vi "ADCP_UI.vi"() -> ()   [LabVIEW 2017]
uses:
  Controls/ADCP_UI/ADCP_UI_Node_Requests.ctl
  Controls/ADCP_UI/ADCP_UI_Parameters.ctl
  Controls/ADCP_UI/ADCP_UI_Queues.ctl
  Controls/ADCP_UI/ADCP_UI_Continuous_Receiver_States.ctl
  Controls/ADCP_UI/ADCP_Queue_Receive_Log_Queue_Element.ctl
  Controls/Packet/Packet.ctl
  Controls/Packet/Packet_Direction.ctl
  Controls/Packet/Packet_Type.ctl
  Controls/Packet/Packet_Priority.ctl
  Controls/Data Packets/Data_Packet.ctl
  Controls/Data Packets/Parameter.ctl
  Controls/Data Packets/Parameter_Data_Type.ctl
  Controls/Data Packets/Data_Packet_Transmit_Mode.ctl
  ADCP_UI_Receive_List_Data_Packets.vi
panel:
  out "Node Requests":T1
  out "Receiver queue size":u32
  out "Receiver Queue Status":enum16{"OK", "EMPTY", "FULL"}(ring)
  out "Network Error Status":T2(ring)
  in  "Stop Application":bool
  in  "Receive Data Packet Log File Path":path
  in  "Transmit Data Packet Log File Path":path
  in  "Remove transmit list frame":bool
  in  "Add transmit list frame":bool
  in  "Transmit List Frame name":string(combo)
  out "Request frames":string[](array[string])
  in  "Remove request frame":bool
  in  "Add request frame":bool
  in  "Request Frame":string(combo)
  in  "Request frames from node":bool
  in  "Enable/disable node":bool
  in  "Get node status":bool
  in  "Reset nodes":bool
  in  "Node names":string(combo)="0"
  in  "Reset node":bool
  in  "Transmit List":string[][](table)
  in  "Receive List":string[][](table)
  in  "Load Symbol File":bool
  in  "Symbol File Path":path=path "F:/Projects/ADCP/LabVIEW/Symbol Files/default.csv"
  in  "Connect/Disconnect":bool
  in  "Baud rate":u32=38400
  in  "COM Port":refnum<visa-resource-name>="COM13"
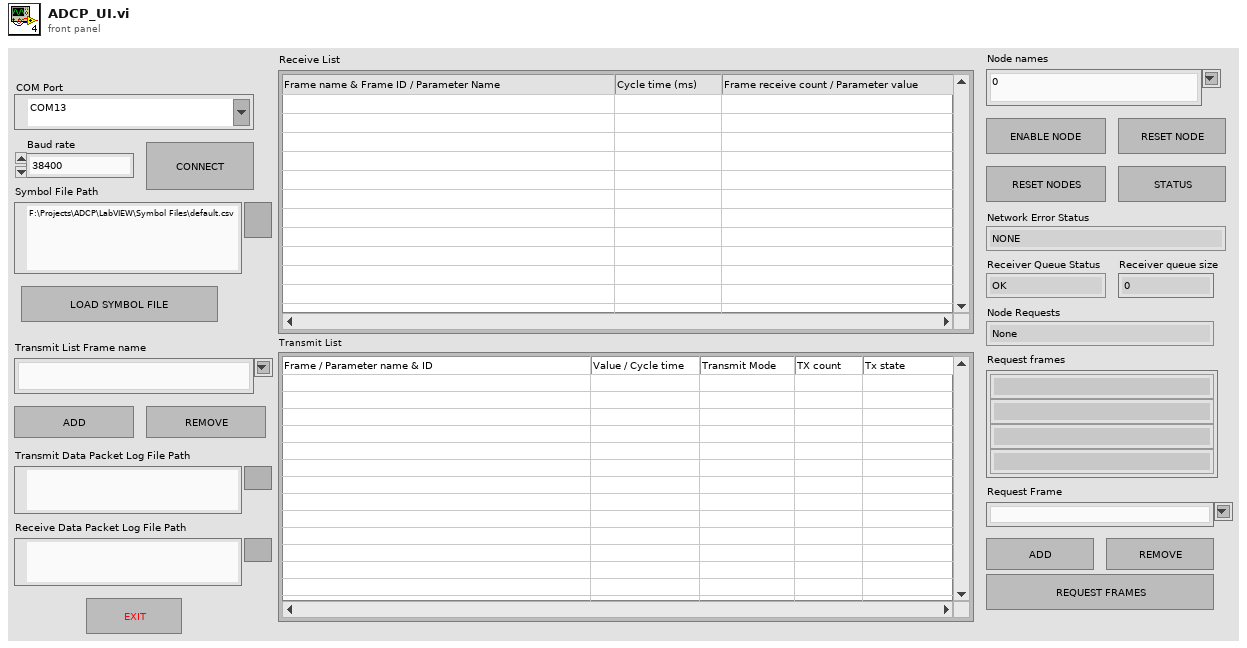
[diagram p1: front panel]
types:
  T1 = typedef "ADCP_UI_Node_Requests.ctl" = enum16{"None", "Open Connection RQST", "Open Connection ACK", "Close Connection RQST", "Close Connection ACK", "Sync/Reset RQST", "Sync/Reset ACK", "Error & Status RQST", "Error & Status ACK", "Remote Request RQST", "Remote Request ACK", "Timeout"}
  T2 = enum16{"NONE", "CONNECTION_ALREADY_OPEN", "CONNECTION_ALREADY_CLOSED", "INVALID_FRAME_REQUEST"}
  T3 = typedef "ADCP_UI_Parameters.ctl" = cluster{"COM Port":refnum<vi>, "Baud rate":refnum<vi>, "Symbol File Path":refnum<vi>, "Receive List":refnum<vi>, "Transmit List":refnum<vi>, "Node names":refnum<vi>, "Request Frame":refnum<vi>, "Request frames":refnum<vi>, "Transmit List Frame name":refnum<vi>, "Transmit Data Packet Log File Path":refnum<vi>, "Receive Data Packet Log File Path":refnum<vi>, "Loop 1 Resume Request":bool, "Loop 1 Pause Request":bool, "Loop 2 Resume Request":bool, "Loop 2 Pause Request":bool, "Loop 3 Resume Request":bool, "Loop 3 Pause Request":bool, "Loop 4 Resume Request":bool, "Loop 4 Pause Request":bool, "Loop 5 Resume Request":bool, "Loop 5 Pause Request":bool, "Loop 6 Resume Request":bool, "Loop 6 Pause Request":bool, "Loop 7 Resume Request":bool, "Loop 7 Pause Request":bool, "Loop 8 Resume Request":bool, "Loop 8 Pause Request":bool, "Exit":refnum<vi>, "Connect/Disconnect":refnum<vi>, "Load Symbol File":refnum<vi>, "Reset node":refnum<vi>, "Reset nodes":refnum<vi>, "Get node status":refnum<vi>, "Enable/disable node":refnum<vi>, "Request frames from node":refnum<vi>, "Remove request frame":refnum<vi>, "Add request frame":refnum<vi>, "Remove transmit list frame":refnum<vi>, "Add transmit list frame":refnum<vi>, "Receiver queue size":refnum<vi>, "Network Error Status":refnum<vi>, "Receiver Queue Status":refnum<vi>, "Node Requests":refnum<vi>, "Queues":T4}
  T4 = typedef "ADCP_UI_Queues.ctl" = cluster{"Continuous Receiver - Getter":refnum<queue>, "Continuous Receiver - Setter":refnum<queue>, "Receive Log":refnum<queue>, "Receive Table":refnum<queue>, "Receive List UI Table Updater":refnum<queue>, "Continuous Transmitter - Getter":refnum<queue>, "Continuous Transmitter - Setter":refnum<queue>, "Transmit Log":refnum<queue>, "Transmit Table":refnum<queue>}
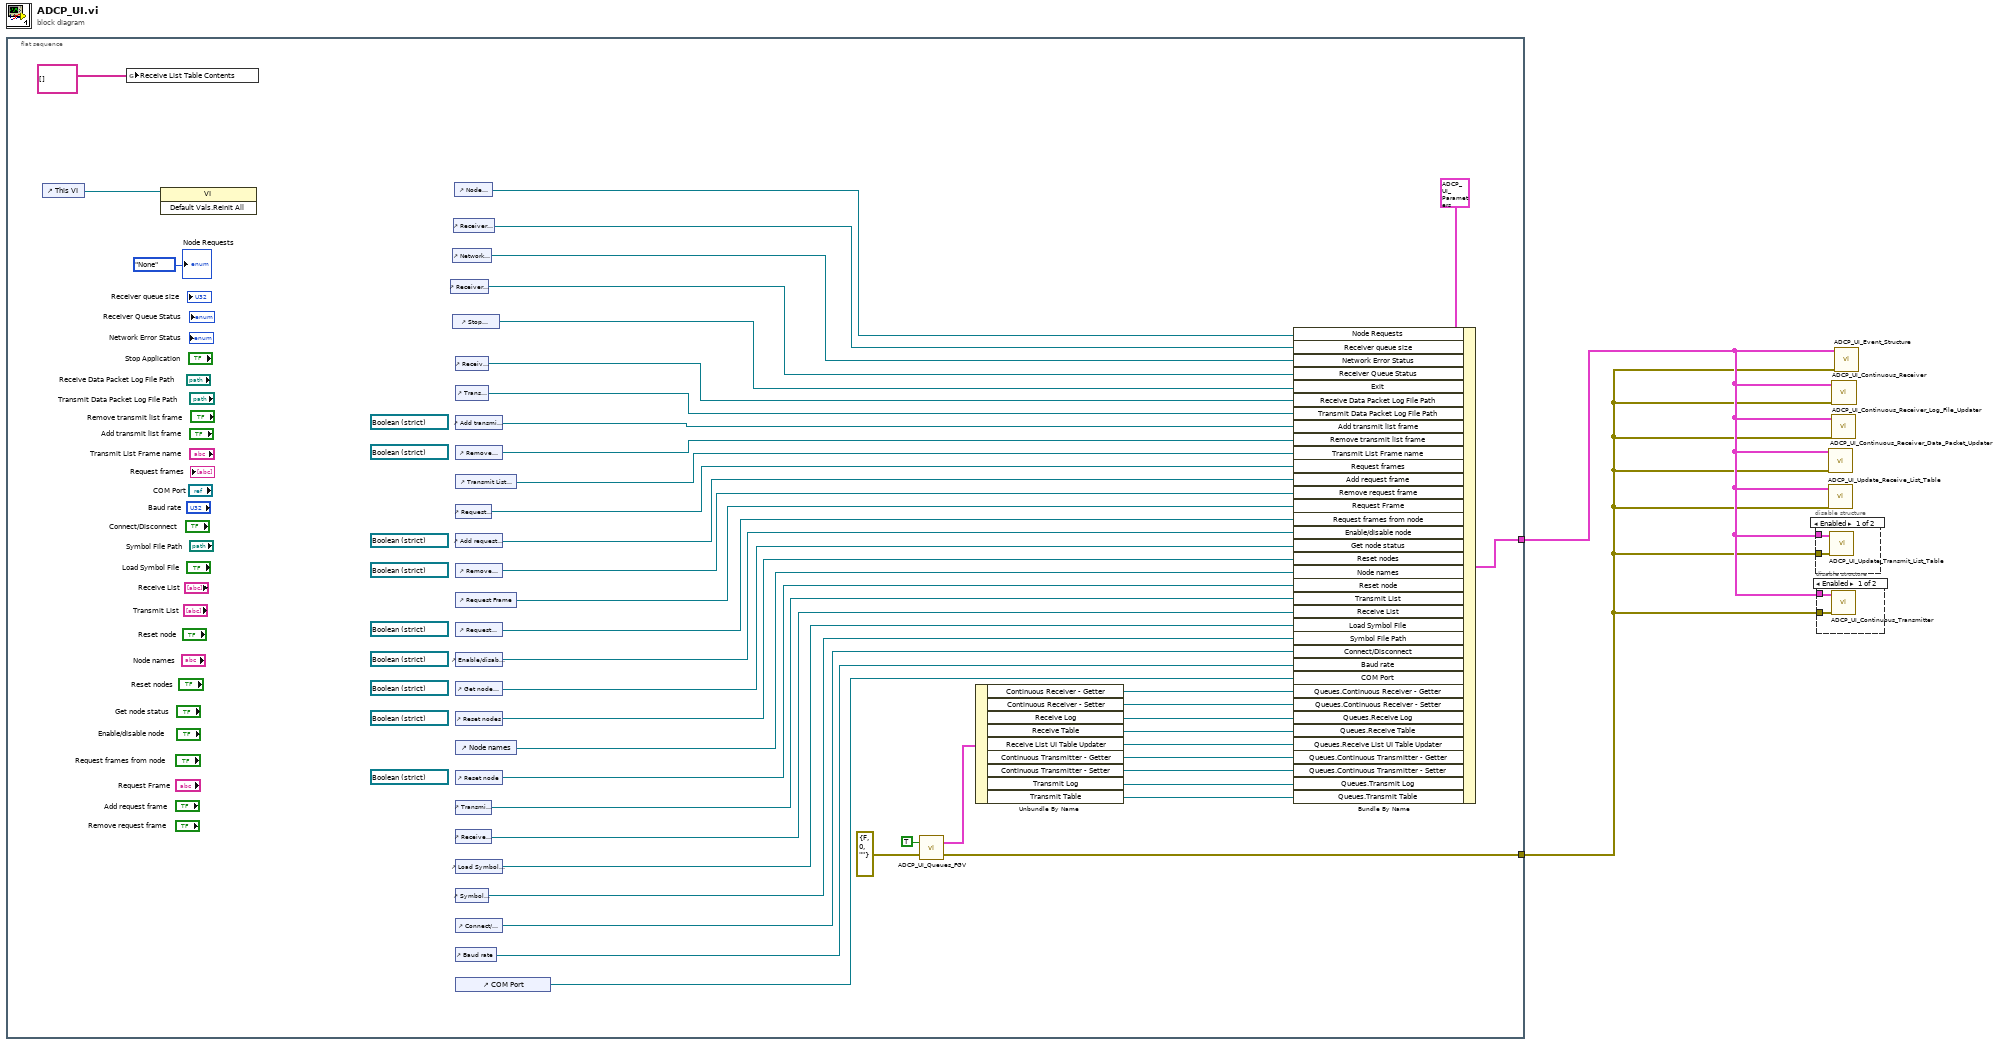
[diagram p0: block diagram]
diagram:
  n1 = flat-sequence {
    tunnel: [w25] -> w2
    tunnel: [w16] -> w1
    frame #0 {
      (unwired) refnum<vi> refnum ("Add transmit list frame")
      (unwired) refnum<vi> refnum ("Remove transmit list frame")
      (unwired) refnum<vi> refnum ("Add request frame")
      (unwired) refnum<vi> refnum ("Remove request frame")
      (unwired) refnum<vi> refnum ("Request frames from node")
      (unwired) refnum<vi> refnum ("Enable/disable node")
      (unwired) refnum<vi> refnum ("Get node status")
      (unwired) refnum<vi> refnum ("Reset nodes")
      (unwired) refnum<vi> refnum ("Reset node")
      n2 = control-ref of="This VI"() -> (w8:refnum<vi>)
      n3 = global write "ADCP_UI_Receive_List_Data_Packets.vi" "Receive List Table Contents"(string[][] []) -> ()
      n4 = invoke class="VI" method="Default Vals.Reinit All"(reference=w8) -> ()  [unwired: 2 in, 3 out]
      n5 = control-ref of="Receiver Queue Status"() -> (w20:refnum<vi>)
      n6 = control-ref of="Stop Application"() -> (w23:refnum<vi>)
      n7 = control-ref of="Network Error Status"() -> (w21:refnum<vi>)
      n8 = control-ref of="Receiver queue size"() -> (w22:refnum<vi>)
      n9 = control-ref of="Node Requests"() -> (w18:refnum<vi>)
      n10 = control-ref of="Receive Data Packet Log File Path"() -> (w46:refnum<vi>)
      n11 = control-ref of="Transmit Data Packet Log File Path"() -> (w45:refnum<vi>)
      n12 = control-ref of="Add transmit list frame"() -> (w24:refnum<vi>)
      n13 = control-ref of="Remove transmit list frame"() -> (w44:refnum<vi>)
      n14 = control-ref of="Transmit List Frame name"() -> (w43:refnum<vi>)
      n15 = control-ref of="Request frames"() -> (w42:refnum<vi>)
      n16 = control-ref of="Add request frame"() -> (w41:refnum<vi>)
      n17 = control-ref of="Remove request frame"() -> (w40:refnum<vi>)
      n18 = control-ref of="Request Frame"() -> (w39:refnum<vi>)
      n19 = control-ref of="Request frames from node"() -> (w38:refnum<vi>)
      n20 = control-ref of="Enable/disable node"() -> (w37:refnum<vi>)
      n21 = control-ref of="Get node status"() -> (w36:refnum<vi>)
      n22 = control-ref of="Reset nodes"() -> (w35:refnum<vi>)
      n23 = control-ref of="Node names"() -> (w34:refnum<vi>)
      n24 = control-ref of="Reset node"() -> (w33:refnum<vi>)
      n25 = control-ref of="Transmit List"() -> (w32:refnum<vi>)
      n26 = control-ref of="Receive List"() -> (w31:refnum<vi>)
      n27 = control-ref of="Load Symbol File"() -> (w30:refnum<vi>)
      n28 = control-ref of="Symbol File Path"() -> (w29:refnum<vi>)
      n29 = control-ref of="Connect/Disconnect"() -> (w28:refnum<vi>)
      n30 = control-ref of="Baud rate"() -> (w27:refnum<vi>)
      n31 = control-ref of="COM Port"() -> (w26:refnum<vi>)
      n32 = call "ADCP_UI_Queues_FGV.vi"("error in (no error)"=errorcluster {"status"=FALSE, "code"=0, "source"=""} ("error constant"), "Initialize ?"=TRUE) -> ("error out"=w16:errorcluster, "Queues"=w14:T4)
      n33 = Unbundle By Name(w14) -> ("Continuous Receiver - Getter"=w13:refnum<queue>, "Continuous Receiver - Setter"=w12:refnum<queue>, "Receive Log"=w11:refnum<queue>, "Receive Table"=w10:refnum<queue>, "Receive List UI Table Updater"=w9:refnum<queue>, "Continuous Transmitter - Getter"=w6:refnum<queue>, "Continuous Transmitter - Setter"=w5:refnum<queue>, "Transmit Log"=w4:refnum<queue>, "Transmit Table"=w3:refnum<queue>)
      n34 = Bundle By Name(cluster=T3 {"COM Port"=refnum, "Baud rate"=refnum, "Symbol File Path"=refnum, "Receive List"=refnum, "Transmit List"=refnum, "Node names"=refnum, "Request Frame"=refnum, "Request frames"=refnum, "Transmit List Frame name"=refnum, "Transmit Data Packet Log File Path"=refnum, "Receive Data Packet Log File Path"=refnum, "Loop 1 Resume Request"=FALSE, "Loop 1 Pause Request"=FALSE, "Loop 2 Resume Request"=FALSE, "Loop 2 Pause Request"=FALSE, "Loop 3 Resume Request"=FALSE, "Loop 3 Pause Request"=FALSE, "Loop 4 Resume Request"=FALSE, "Loop 4 Pause Request"=FALSE, "Loop 5 Resume Request"=FALSE, "Loop 5 Pause Request"=FALSE, "Loop 6 Resume Request"=FALSE, "Loop 6 Pause Request"=FALSE, "Loop 7 Resume Request"=FALSE, "Loop 7 Pause Request"=FALSE, "Loop 8 Resume Request"=FALSE, "Loop 8 Pause Request"=FALSE, "Exit"=refnum, "Connect/Disconnect"=refnum, "Load Symbol File"=refnum, "Reset node"=refnum, "Reset nodes"=refnum, "Get node status"=refnum, "Enable/disable node"=refnum, "Request frames from node"=refnum, "Remove request frame"=refnum, "Add request frame"=refnum, "Remove transmit list frame"=refnum, "Add transmit list frame"=refnum, "Receiver queue size"=refnum, "Network Error Status"=refnum, "Receiver Queue Status"=refnum, "Node Requests"=refnum, "Queues"={"Continuous Receiver - Getter"=refnum, "Continuous Receiver - Setter"=refnum, "Receive Log"=refnum, "Receive Table"=refnum, "Receive List UI Table Updater"=refnum, "Continuous Transmitter - Getter"=refnum, "Continuous Transmitter - Setter"=refnum, "Transmit Log"=refnum, "Transmit Table"=refnum}} ("ADCU_GUI References"), "Node Requests"=w18, "Receiver queue size"=w22, "Network Error Status"=w21, "Receiver Queue Status"=w20, "Exit"=w23, "Receive Data Packet Log File Path"=w46, "Transmit Data Packet Log File Path"=w45, "Add transmit list frame"=w24, "Remove transmit list frame"=w44, "Transmit List Frame name"=w43, "Request frames"=w42, "Add request frame"=w41, "Remove request frame"=w40, "Request Frame"=w39, "Request frames from node"=w38, "Enable/disable node"=w37, "Get node status"=w36, "Reset nodes"=w35, "Node names"=w34, "Reset node"=w33, "Transmit List"=w32, "Receive List"=w31, "Load Symbol File"=w30, "Symbol File Path"=w29, "Connect/Disconnect"=w28, "Baud rate"=w27, "COM Port"=w26, "Queues.Continuous Receiver - Getter"=w13, "Queues.Continuous Receiver - Setter"=w12, "Queues.Receive Log"=w11, "Queues.Receive Table"=w10, "Queues.Receive List UI Table Updater"=w9, "Queues.Continuous Transmitter - Getter"=w6, "Queues.Continuous Transmitter - Setter"=w5, "Queues.Transmit Log"=w4, "Queues.Transmit Table"=w3) -> (w25:T3)
      "Node Requests" <- ADCP_UI_Node_Requests."None" ("Node Requests")
    }
  }
  n35 = disable-structure shown="Enabled" {
    disable-tunnel: w2 -> [w49 _]
    disable-tunnel: w1 -> [w48 _]
    frame Enabled {
      n36 = call "ADCP_UI_Update_Transmit_List_Table.vi"("error in (no error)"=w48, "ADCU_GUI References"=w49) -> ()  [unwired: 10 in]
    }
    frame Disabled {
    }
  }
  n37 = disable-structure shown="Enabled" {
    disable-tunnel: w2 -> [w51 _]
    disable-tunnel: w1 -> [w50 _]
    frame Enabled {
      n38 = call "ADCP_UI_Continuous_Transmitter.vi"("error in (no error)"=w50, "ADCU_GUI References"=w51) -> ()  [unwired: 10 in]
    }
    frame Disabled {
    }
  }
  n39 = call "ADCP_UI_Update_Receive_List_Table.vi"("error in (no error)"=w1, "ADCU_GUI References"=w2) -> ()  [unwired: 10 in]
  n40 = call "ADCP_UI_Continuous_Receiver_Data_Packet_Updater.vi"("error in (no error)"=w1, "ADCU_GUI References"=w2) -> ()  [unwired: 10 in]
  n41 = call "ADCP_UI_Continuous_Receiver_Log_File_Updater.vi"("error in (no error)"=w1, "ADCU_GUI References"=w2) -> ()  [unwired: 10 in]
  n42 = call "ADCP_UI_Continuous_Receiver.vi"("error in (no error)"=w1, "ADCU_GUI References"=w2) -> ()  [unwired: 10 in]
  n43 = call "ADCP_UI_Event_Structure.vi"("error in (no error)"=w1, "ADCU_GUI References"=w2) -> ()  [unwired: 10 in]
